vi "Compute slopes from compensate values.vi"(0 "SAVE_Aberrations Filter in":T4, 5 "FilteredSlopesX in":dbl[][](array[numeric]), 7 "FilteredSlopesY in":dbl[][](array[numeric]), 9 "Pupil":i32[][](array[numeric]), 11 "Dimensions_um":T1, 12 "SlopesX_fitting":cluster{"a":dbl, "b":dbl, "c":dbl}, 13 "SlopesY_fitting":cluster{"a":dbl, "b":dbl, "c":dbl}, 14 "Delta_um":T3) -> (6 "FilteredSlopesX out":dbl[][](array[numeric]), 8 "FilteredSlopesY out":dbl[][](array[numeric]))   [LabVIEW 2020]
uses:
  Point2Df.ctl
  General dimensions definition.ctl
  Point2D.ctl
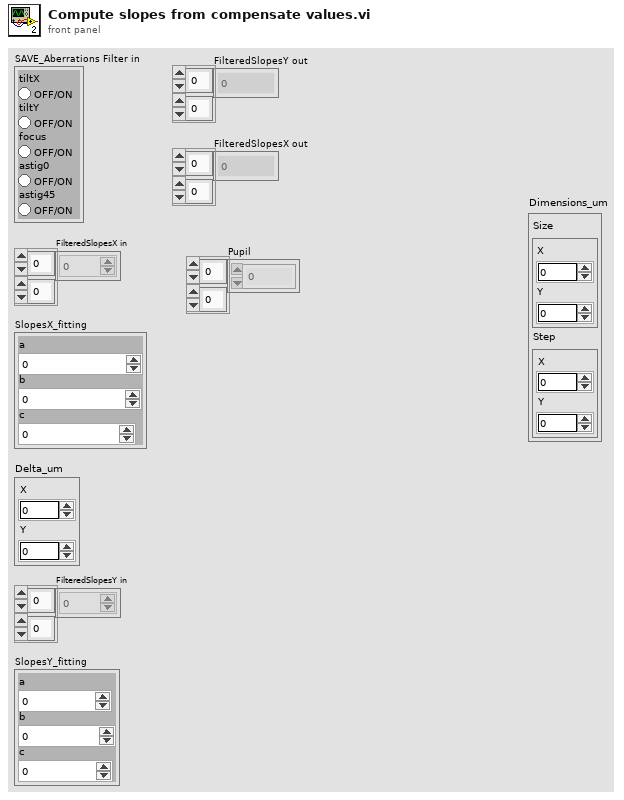
[diagram p1: front panel]
types:
  T1 = typedef "General dimensions definition.ctl" = cluster{"Size":T2, "Step":T3}
  T2 = typedef "Point2D.ctl" = cluster{"X":u32, "Y":u32}
  T3 = typedef "Point2Df.ctl" = cluster{"X":sgl, "Y":sgl}
  T4 = cluster{"tiltX":bool, "tiltY":bool, "focus":bool, "astig0":bool, "astig45":bool}
  T5 = cluster{"ax":dbl, "bx":dbl, "cx":dbl, "ay":dbl, "by":dbl, "cy":dbl, "Delta":T3}
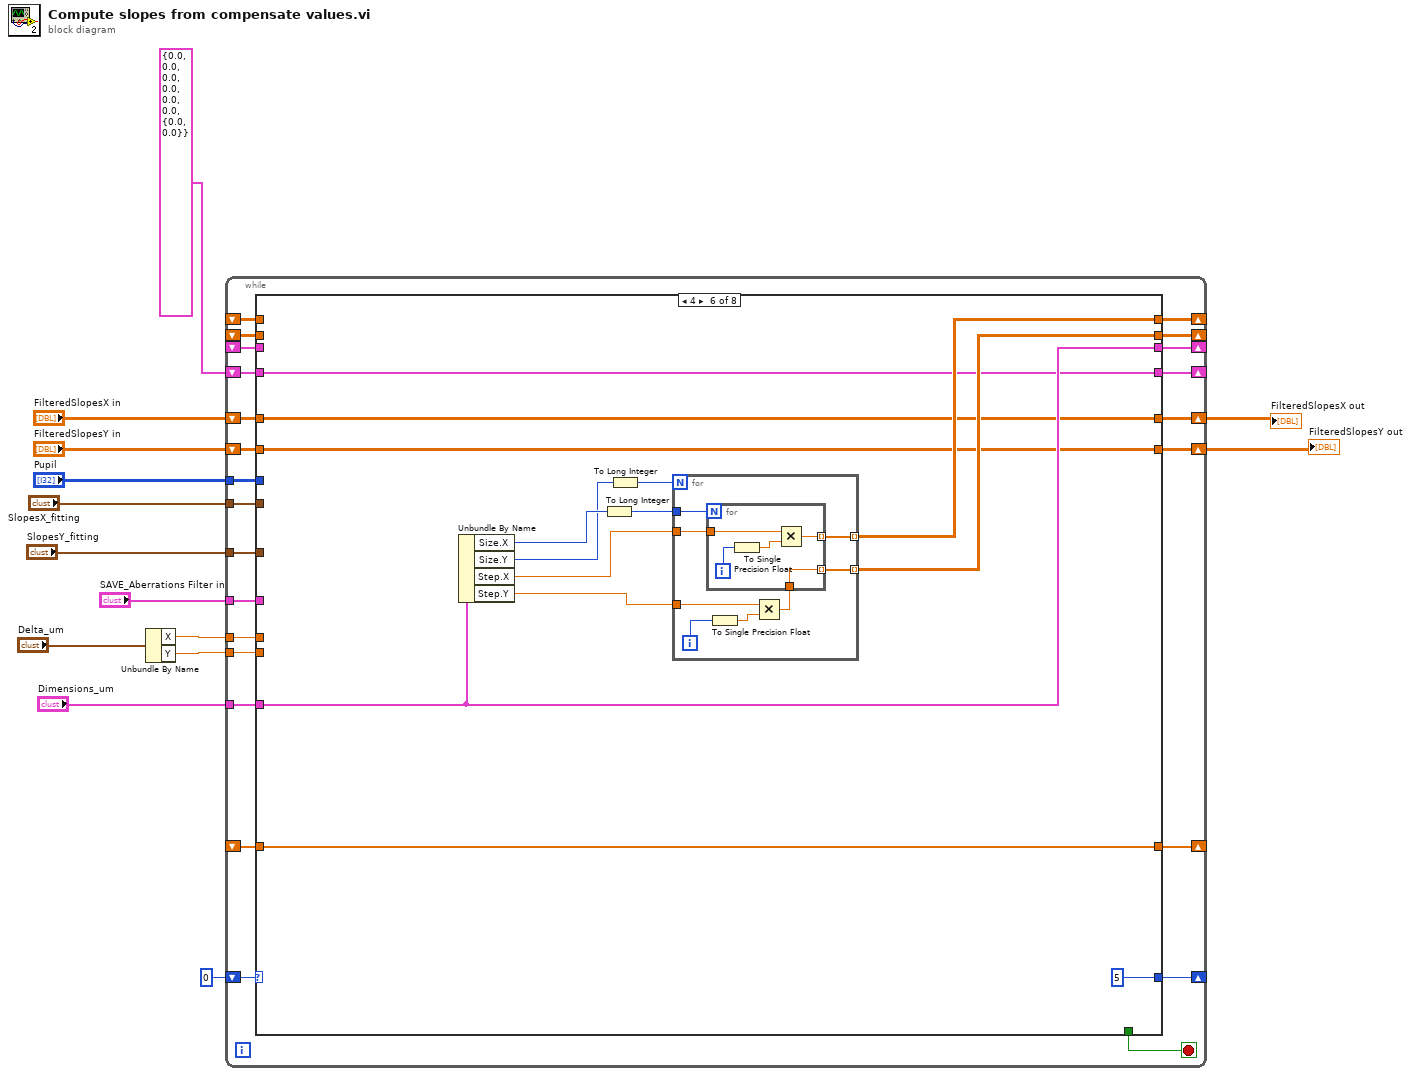
[diagram p0: block diagram]
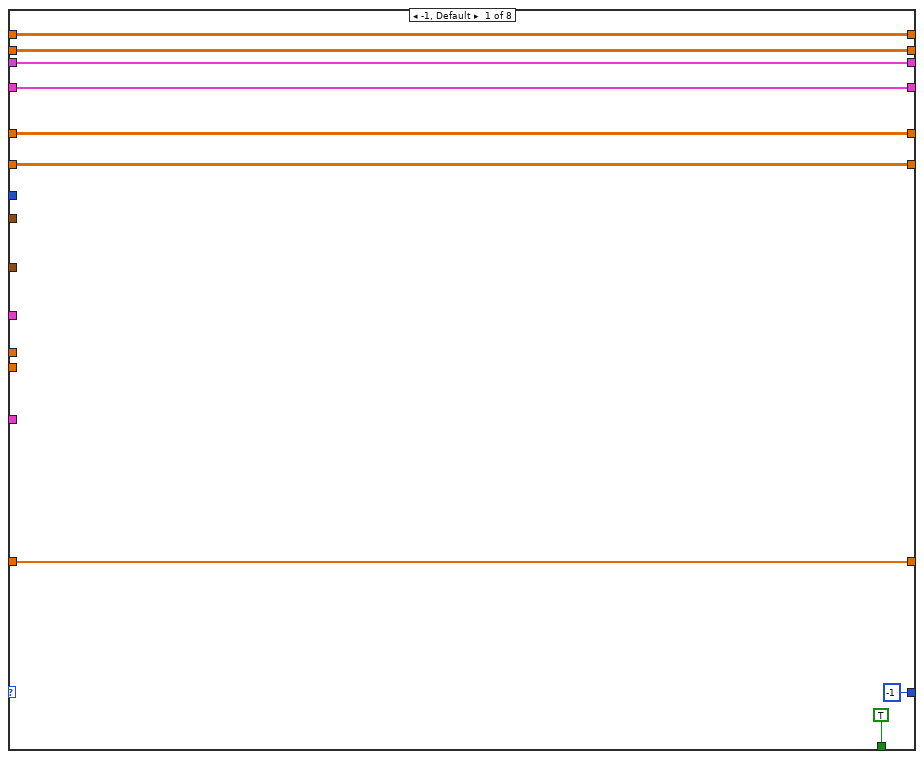
[diagram p2: hidden frame]
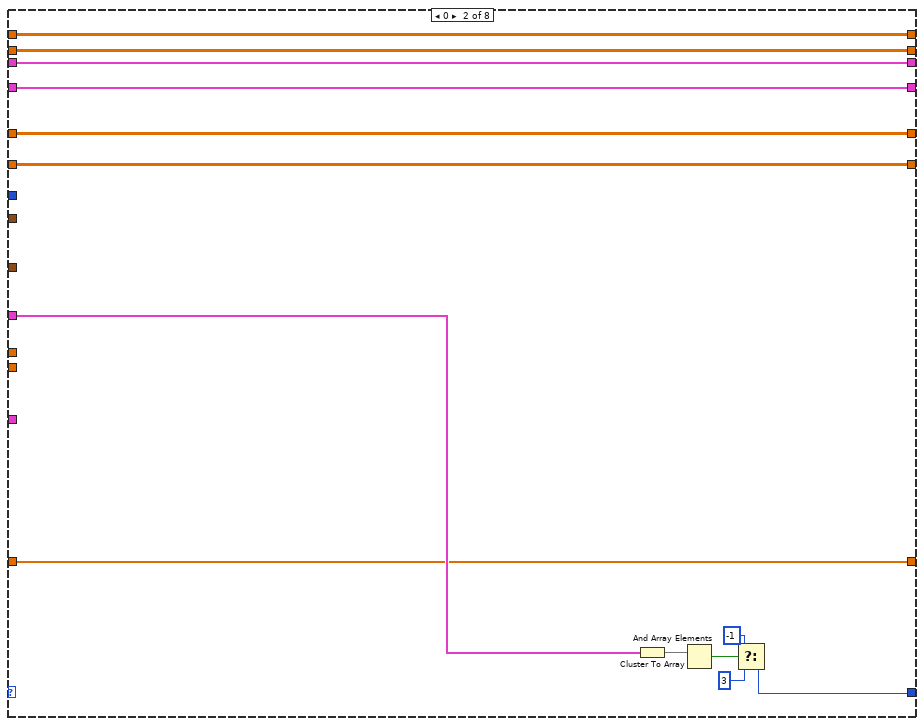
[diagram p3: hidden frame]
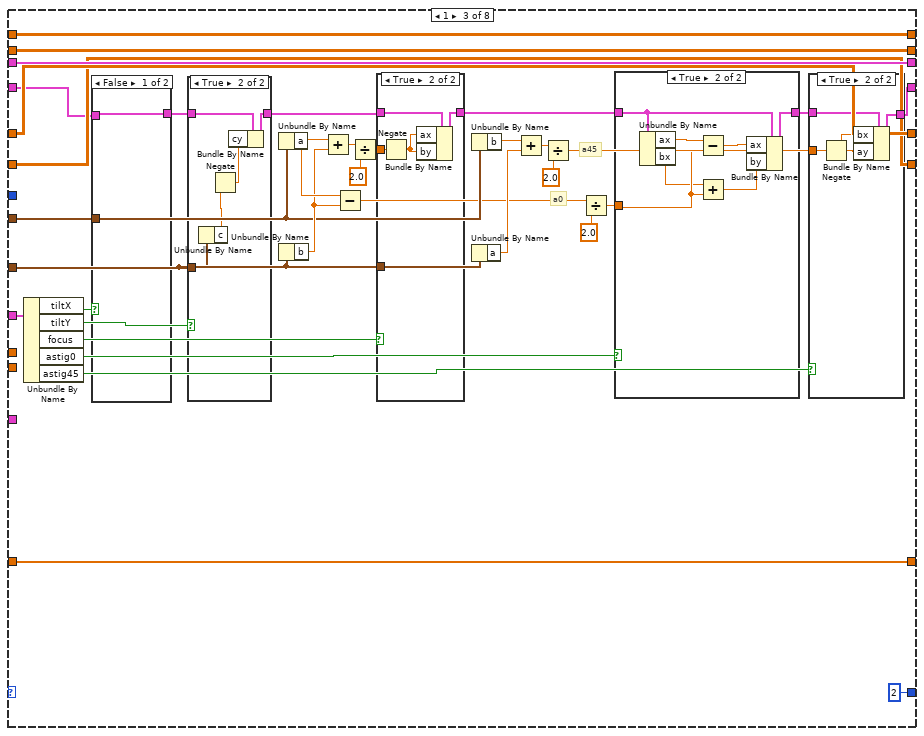
[diagram p4: hidden frame]
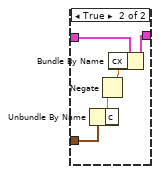
[diagram p9: hidden frame]
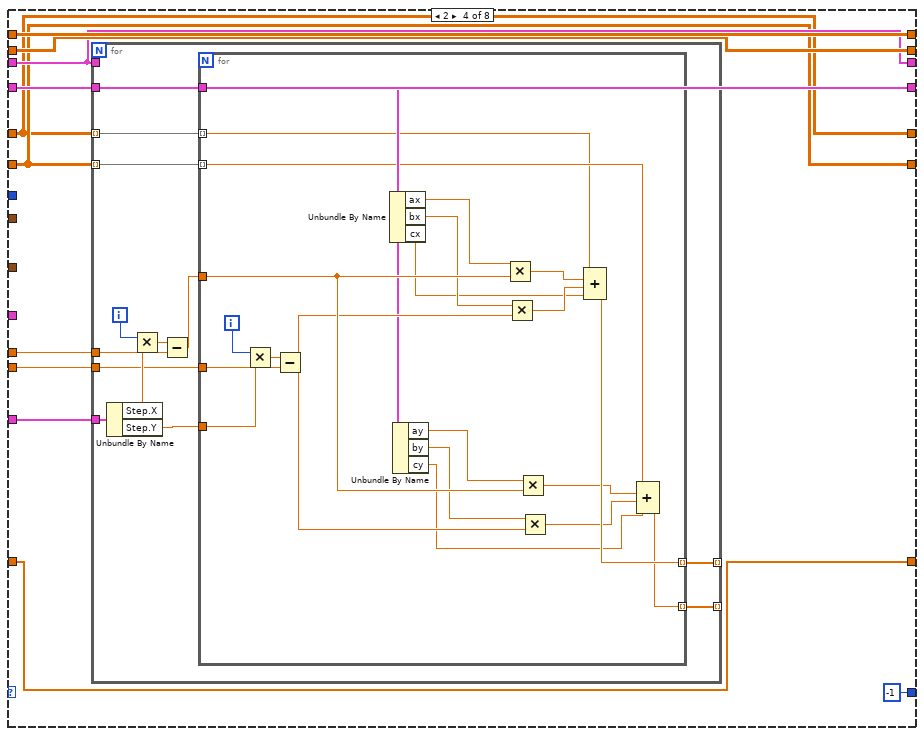
[diagram p10: hidden frame]
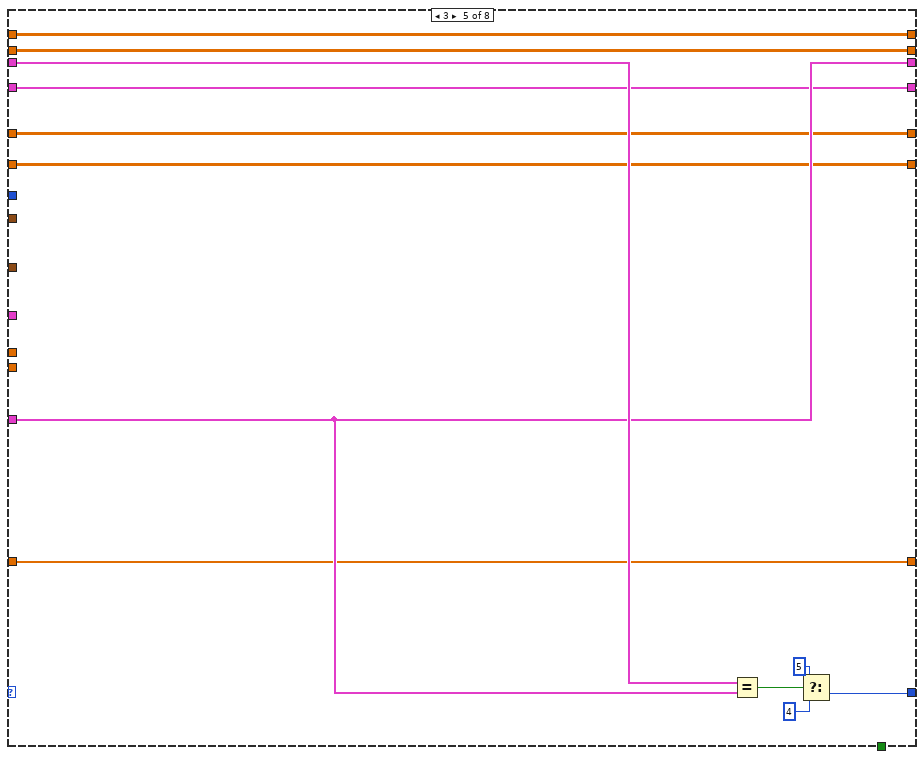
[diagram p11: hidden frame]
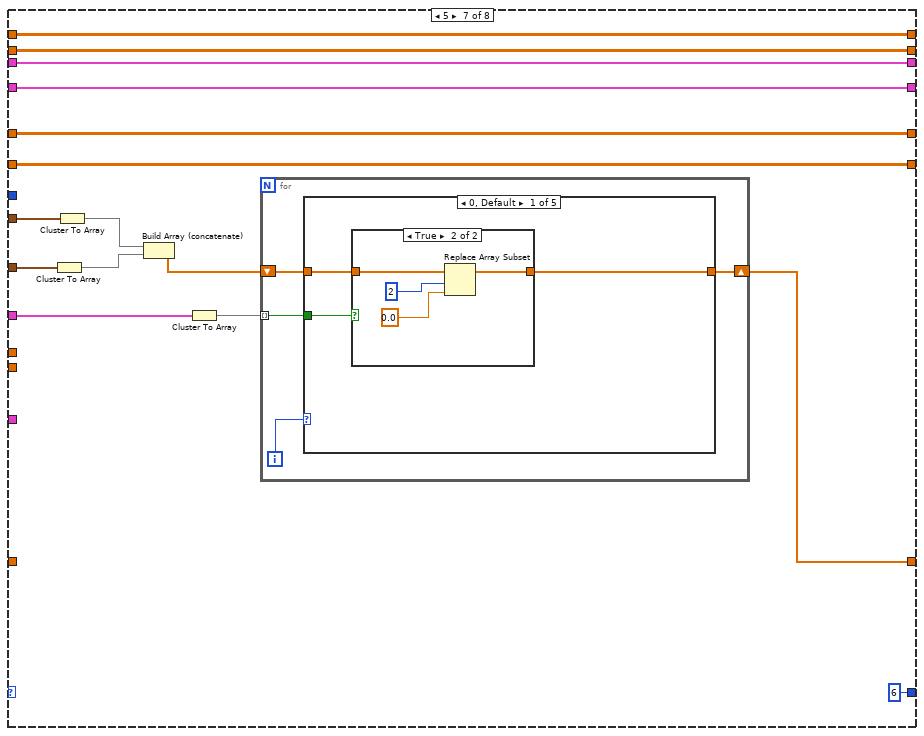
[diagram p12: hidden frame]
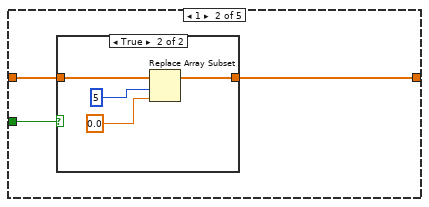
[diagram p14: hidden frame]
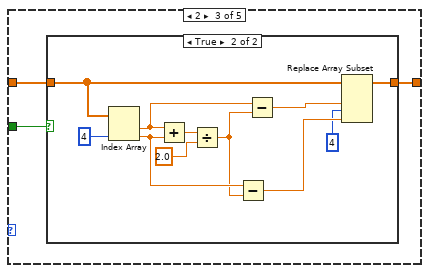
[diagram p16: hidden frame]
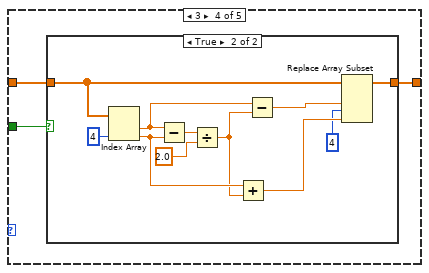
[diagram p18: hidden frame]
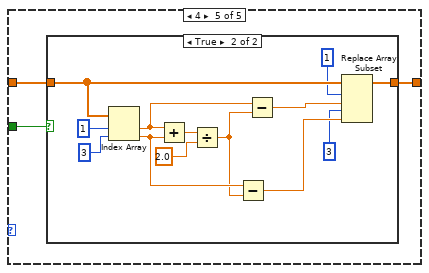
[diagram p20: hidden frame]
diagram:
  n1 = Unbundle By Name("Delta_um") -> ("X"=w3:sgl, "Y"=w2:sgl)
  n2 = while {
    tunnel: "SAVE_Aberrations Filter in" -> [w38]
    tunnel: "SlopesX_fitting" -> [w37]
    tunnel: "SlopesY_fitting" -> [w36]
    shift-right: [w33] -> _
    shift-left: 0 -> [w35]
    shift-right: [w19] -> w6
    shift-left: "FilteredSlopesX in" -> [w21]
    shift-right: [w18] -> w12
    shift-left: "FilteredSlopesY in" -> [w20]
    shift-right: [w34] -> _
    shift-left: T5 {"ax"=0.0, "bx"=0.0, "cx"=0.0, "ay"=0.0, "by"=0.0, "cy"=0.0, "Delta"={"X"=0.0, "Y"=0.0}} -> [w15]
    tunnel: "Dimensions_um" -> [w31]
    tunnel: w3 -> [w30]
    tunnel: w2 -> [w29]
    shift-right: [w27] -> _
    shift-left: _ -> [w28]
    shift-right: [w25] -> _
    shift-left: _ -> [w24]
    shift-right: [w26] -> _
    shift-left: _ -> [w23]
    shift-right: [w22] -> _
    shift-left: _ -> [w17]
    tunnel: "Pupil" -> [w16]
    stop <- w32 stop-if-true
    n3 = case shown="4" w35 {
      tunnel: w38 -> [_ w59 w94 _ _ _ w218 _]
      tunnel: w37 -> [_ _ w76 _ _ _ w217 _]
      tunnel: w36 -> [_ _ w77 _ _ _ w216 _]
      tunnel: [w39 w48 w61 w127 w170 w182 w209 w291] -> w34
      tunnel: [-1 w55 2 -1 w178 5 6 -1] -> w33
      tunnel: [TRUE _ _ _ _ _ _ _] -> w32
      tunnel: w31 -> [_ _ _ w135 w176 w189 _ _]
      tunnel: w30 -> [_ _ _ w134 _ _ _ w294]
      tunnel: w29 -> [_ _ _ w133 _ _ _ w292]
      tunnel: w28 -> [w43 w52 w66 w128 w177 _ w220 w302]
      tunnel: [w43 w52 w66 w128 w176 w189 w220 w302] -> w27
      tunnel: [w44 w53 w67 w130 w174 w188 w221 w293] -> w26
      tunnel: [w45 w54 w68 w131 w175 w187 w222 w297] -> w25
      tunnel: w24 -> [w45 w54 w68 w131 w175 _ w222 w297]
      tunnel: w23 -> [w44 w53 w67 w130 w174 _ w221 w293]
      tunnel: [w40 w49 w63 w129 w171 w183 w212 w295] -> w22
      tunnel: w21 -> [w42 w51 w65 w125 w173 w185 w211 w301]
      tunnel: w20 -> [w41 w50 w64 w126 w172 w184 w210 w300]
      tunnel: [w42 w51 w65 w125 w173 w185 w211 w299] -> w19
      tunnel: [w41 w50 w64 w126 w172 w184 w210 w298] -> w18
      tunnel: w17 -> [w40 w49 w63 w129 w171 w183 _ w295]
      tunnel: w16 -> [_ _ _ _ _ _ _ w296]
      tunnel: w15 -> [w39 w48 w62 w127 w170 w182 w209 w291]
      frame -1, Default {
      }
      frame 0 {
        n4 = Cluster To Array(cluster=w59) -> (array=w60:bool[])
        n5 = And Array Elements(Boolean array=w60) -> (logical AND=w57:bool)
        n6 = Select(t=-1, s=w57, f=3) -> (s? t:f=w55:i32)
      }
      frame 1 {
        # "a45"
        # "a0"
        n7 = Unbundle By Name(w94) -> ("tiltX"=w93:bool, "tiltY"=w91:bool, "focus"=w86:bool, "astig0"=w85:bool, "astig45"=w72:bool)
        n8 = case shown="False" w93 {
          tunnel: [w119 w124] -> w92
          tunnel: w76 -> [_ w122]
          tunnel: w62 -> [w119 w120]
          frame False {
          }
          frame True {
            n9 = Unbundle By Name(w122) -> ("c"=w123:dbl)
            n10 = Negate(x=w123) -> (-x=w121:dbl)
            n11 = Bundle By Name(cluster=w120, "cx"=w121) -> (w124:T5)
          }
        }
        n12 = case shown="True" w91 {
          tunnel: w92 -> [w113 w118]
          tunnel: [w113 w117] -> w90
          tunnel: w77 -> [_ w116]
          frame False {
          }
          frame True {
            n13 = Unbundle By Name(w116) -> ("c"=w115:dbl)
            n14 = Negate(x=w115) -> (-x=w114:dbl)
            n15 = Bundle By Name(cluster=w118, "cy"=w114) -> (w117:T5)
          }
        }
        n16 = Unbundle By Name(w76) -> ("a"=w83:dbl)
        n17 = Unbundle By Name(w77) -> ("b"=w82:dbl)
        n18 = Add(x=w83, y=w82) -> (x+y=w88:dbl)
        n19 = Subtract(x=w83, y=w82) -> (x-y=w74:dbl)
        n20 = Divide(x=w88, y=2.0) -> (x/y=w87:dbl)
        n21 = case shown="True" w86 {
          tunnel: w90 -> [w108 w112]
          tunnel: [w108 w111] -> w84
          tunnel: w77 -> [_ _]
          tunnel: w87 -> [_ w110]
          frame False {
          }
          frame True {
            n22 = Negate(x=w110) -> (-x=w109:dbl)
            n23 = Bundle By Name(cluster=w112, "ax"=w109, "by"=w109) -> (w111:T5)
          }
        }
        n24 = Unbundle By Name(w76) -> ("b"=w80:dbl)
        n25 = Unbundle By Name(w77) -> ("a"=w81:dbl)
        n26 = Add(x=w80, y=w81) -> (x+y=w79:dbl)
        n27 = Divide(x=w79, y=2.0) -> (x/y=w71:dbl)
        n28 = Divide(x=w74, y=2.0) -> (x/y=w73:dbl)
        n29 = case shown="True" w85 {
          tunnel: w84 -> [w100 w106]
          tunnel: [w100 w107] -> w70
          tunnel: w73 -> [_ w104]
          frame False {
          }
          frame True {
            n30 = Unbundle By Name(w106) -> ("ax"=w102:dbl, "bx"=w101:dbl)
            n31 = Subtract(x=w102, y=w104) -> (x-y=w105:dbl)
            n32 = Add(x=w101, y=w104) -> (x+y=w103:dbl)
            n33 = Bundle By Name(cluster=w106, "ax"=w105, "by"=w103) -> (w107:T5)
          }
        }
        n34 = case shown="True" w72 {
          tunnel: w71 -> [_ w98]
          tunnel: w70 -> [w95 w99]
          tunnel: [w95 w96] -> w61
          frame False {
          }
          frame True {
            n35 = Negate(x=w98) -> (-x=w97:dbl)
            n36 = Bundle By Name(cluster=w99, "bx"=w97, "ay"=w97) -> (w96:T5)
          }
        }
      }
      frame 2 {
        n37 = for {
          tunnel: w135 -> [w147]
          tunnel: w134 -> [w144]
          tunnel: w133 -> [w142]
          tunnel: [w140] -> _ mode=indexing
          tunnel: [w139] -> _ mode=indexing
          tunnel: w128 -> [_]
          tunnel: w127 -> [w138]
          tunnel: w126 -> [w137] mode=indexing
          tunnel: w125 -> [w136] mode=indexing
          i -> [w148]
          n38 = Unbundle By Name(w147) -> ("Step.X"=w146:sgl, "Step.Y"=w143:sgl)
          n39 = Multiply(x=w148, y=w146) -> (x*y=w145:sgl)
          n40 = Subtract(x=w145, y=w144) -> (x-y=w141:sgl)
          n41 = for {
            tunnel: w143 -> [w167]
            tunnel: w142 -> [w166]
            tunnel: w141 -> [w160]
            tunnel: [w163] -> w140 mode=indexing
            tunnel: [w158] -> w139 mode=indexing
            tunnel: w138 -> [w157]
            tunnel: w137 -> [w150] mode=indexing
            tunnel: w136 -> [w149] mode=indexing
            i -> [w168]
            n42 = Multiply(x=w168, y=w167) -> (x*y=w169:sgl)
            n43 = Subtract(x=w169, y=w166) -> (x-y=w159:sgl)
            n44 = Unbundle By Name(w157) -> ("ax"=w156:dbl, "bx"=w155:dbl, "cx"=w154:dbl)
            n45 = Unbundle By Name(w157) -> ("ay"=w153:dbl, "by"=w152:dbl, "cy"=w151:dbl)
            n46 = Multiply(x=w156, y=w160) -> (x*y=w165:dbl)
            n47 = Multiply(x=w155, y=w159) -> (x*y=w164:dbl)
            n48 = Multiply(x=w153, y=w160) -> (x*y=w161:dbl)
            n49 = Multiply(x=w152, y=w159) -> (x*y=w162:dbl)
            n50 = Compound Arithmetic op=ADD(w149, w165, w164, w154) -> (w163:dbl)
            n51 = Compound Arithmetic op=ADD(w150, w161, w162, w151) -> (w158:dbl)
          }
        }
      }
      frame 3 {
        n52 = Equal?(x=w177, y=w176) -> (x = y?=w179:bool)
        n53 = Select(t=5, s=w179, f=4) -> (s? t:f=w178:i32)
      }
      frame 4 {
        n54 = Unbundle By Name(w189) -> ("Size.X"=w195:u32, "Size.Y"=w192:u32, "Step.X"=w193:sgl, "Step.Y"=w190:sgl)
        n55 = To Long Integer(number=w195) -> (32bit integer=w194:i32)
        n56 = To Long Integer(number=w192) -> (32bit integer=w191:i32)
        n57 = for {
          N: w191 -> [_]
          tunnel: w194 -> [w203]
          tunnel: w193 -> [w202]
          tunnel: [w201] -> w187 mode=indexing
          tunnel: w190 -> [w198]
          tunnel: [w196] -> w188 mode=indexing
          i -> [w199]
          n58 = To Single Precision Float(number=w199) -> (single precision float=w200:sgl)
          n59 = Multiply(x=w198, y=w200) -> (x*y=w197:sgl)
          n60 = for {
            N: w203 -> [_]
            tunnel: w202 -> [w208]
            tunnel: [w205] -> w201 mode=indexing
            tunnel: w197 -> [w204]
            tunnel: [w204] -> w196 mode=indexing
            i -> [w207]
            n61 = To Single Precision Float(number=w207) -> (single precision float=w206:sgl)
            n62 = Multiply(x=w208, y=w206) -> (x*y=w205:sgl)
          }
        }
      }
      frame 5 {
        n63 = Cluster To Array(cluster=w216) -> (array=w214:dbl[])
        n64 = Cluster To Array(cluster=w217) -> (array=w215:dbl[])
        n65 = Build Array (concatenate)(w215, w214) -> (w213:dbl[])
        n66 = Cluster To Array(cluster=w218) -> (array=w219:bool[])
        n67 = for {
          tunnel: w219 -> [w227] mode=indexing
          shift-right: [w225] -> w212
          shift-left: w213 -> [w226]
          i -> [w224]
          n68 = case shown="0, Default" w224 {
            tunnel: w227 -> [w230 w238 w246 w261 w276]
            tunnel: w226 -> [w229 w237 w245 w260 w275]
            tunnel: [w228 w236 w244 w259 w274] -> w225
            frame 0, Default {
              n69 = case shown="True" w230 {
                tunnel: w229 -> [w231 w235]
                tunnel: [w231 w234] -> w228
                frame False {
                }
                frame True {
                  n70 = Replace Array Subset(array=w235, new element=sgl 0.0 ("new element/subarray"), index=2) -> (w234:dbl[])
                }
              }
            }
            frame 1 {
              n71 = case shown="True" w238 {
                tunnel: w237 -> [w239 w243]
                tunnel: [w239 w242] -> w236
                frame False {
                }
                frame True {
                  n72 = Replace Array Subset(array=w243, new element=sgl 0.0 ("new element/subarray"), index=5) -> (w242:dbl[])
                }
              }
            }
            frame 2 {
              n73 = case shown="True" w246 {
                tunnel: w245 -> [w247 w248]
                tunnel: [w247 w258] -> w244
                frame False {
                }
                frame True {
                  n74 = Index Array(array=w248, index #2=4 ("index")) -> (element #1=w254:dbl, element #2=w253:dbl)  [unwired: 1 in]
                  n75 = Add(x=w254, y=w253) -> (x+y=w256:dbl)
                  n76 = Divide(x=w256, y=sgl 2.0) -> (x/y=w252:dbl)
                  n77 = Subtract(x=w253, y=w252) -> (x-y=w250:dbl)
                  n78 = Subtract(x=w254, y=w252) -> (x-y=w251:dbl)
                  n79 = Replace Array Subset(array=w248, new element #1=w251, new element #2=w250, index #2=4 ("index")) -> (w258:dbl[])  [unwired: 1 in]
                }
              }
            }
            frame 3 {
              n80 = case shown="True" w261 {
                tunnel: w260 -> [w262 w263]
                tunnel: [w262 w273] -> w259
                frame False {
                }
                frame True {
                  n81 = Index Array(array=w263, index #2=4 ("index")) -> (element #1=w269:dbl, element #2=w268:dbl)  [unwired: 1 in]
                  n82 = Subtract(x=w269, y=w268) -> (x-y=w271:dbl)
                  n83 = Divide(x=w271, y=sgl 2.0) -> (x/y=w267:dbl)
                  n84 = Add(x=w268, y=w267) -> (x+y=w265:dbl)
                  n85 = Subtract(x=w269, y=w267) -> (x-y=w266:dbl)
                  n86 = Replace Array Subset(array=w263, new element #1=w266, new element #2=w265, index #2=4 ("index")) -> (w273:dbl[])  [unwired: 1 in]
                }
              }
            }
            frame 4 {
              n87 = case shown="True" w276 {
                tunnel: w275 -> [w277 w280]
                tunnel: [w277 w290] -> w274
                frame False {
                }
                frame True {
                  n88 = Index Array(array=w280, index #1=1 ("index"), index #2=3 ("index")) -> (element #1=w286:dbl, element #2=w285:dbl)
                  n89 = Add(x=w286, y=w285) -> (x+y=w288:dbl)
                  n90 = Divide(x=w288, y=sgl 2.0) -> (x/y=w284:dbl)
                  n91 = Subtract(x=w285, y=w284) -> (x-y=w282:dbl)
                  n92 = Subtract(x=w286, y=w284) -> (x-y=w283:dbl)
                  n93 = Replace Array Subset(array=w280, new element #1=w283, index #1=1 ("index"), new element #2=w282, index #2=3 ("index")) -> (w290:dbl[])
                }
              }
            }
          }
        }
      }
      frame 6 {
        n94 = for {
          tunnel: w301 -> [w313] mode=indexing
          tunnel: w300 -> [w312] mode=indexing
          tunnel: w296 -> [w311] mode=indexing
          tunnel: w295 -> [w310]
          tunnel: [w309] -> w299 mode=indexing
          tunnel: [w308] -> w298 mode=indexing
          tunnel: w297 -> [w307] mode=indexing
          tunnel: w294 -> [w306]
          tunnel: w293 -> [w305] mode=indexing
          tunnel: w292 -> [w304]
          n95 = for {
            tunnel: w313 -> [w322] mode=indexing
            tunnel: w312 -> [w320] mode=indexing
            tunnel: w311 -> [w323] mode=indexing
            tunnel: w310 -> [w321]
            tunnel: [w319] -> w309 mode=indexing
            tunnel: [w318] -> w308 mode=indexing
            tunnel: w307 -> [w317] mode=indexing
            tunnel: w306 -> [w316]
            tunnel: w305 -> [w315] mode=indexing
            tunnel: w304 -> [w314]
            n96 = case shown="1" w323 {
              tunnel: w322 -> [_ w341]
              tunnel: w321 -> [_ w347]
              tunnel: w320 -> [_ w339]
              tunnel: [w324 w332] -> w319
              tunnel: [w324 w331] -> w318
              tunnel: w317 -> [_ w330]
              tunnel: w316 -> [_ w329]
              tunnel: w315 -> [_ w327]
              tunnel: w314 -> [_ w326]
              frame 0, Default {
                w324 = sgl nan
              }
              frame 1 {
                n97 = Subtract(x=w327, y=w326) -> (x-y=w325:sgl)
                n98 = Subtract(x=w330, y=w329) -> (x-y=w328:sgl)
                n99 = Index Array(array=w347) -> (element #1=w346:dbl, element #2=w345:dbl, element #3=w342:dbl, element #4=w336:dbl, element #5=w335:dbl, element #6=w334:dbl)  [unwired: 6 in]
                n100 = Multiply(x=w328, y=w336) -> (x*y=w338:dbl)
                n101 = Multiply(x=w325, y=w335) -> (x*y=w337:dbl)
                n102 = Multiply(x=w328, y=w346) -> (x*y=w343:dbl)
                n103 = Multiply(x=w325, y=w345) -> (x*y=w344:dbl)
                n104 = Compound Arithmetic op=ADD(w338, w337, w334) -> (w333:dbl)
                n105 = Compound Arithmetic op=ADD(w343, w344, w342) -> (w340:dbl)
                n106 = Add(x=w341, y=w340) -> (x+y=w332:dbl)
                n107 = Add(x=w339, y=w333) -> (x+y=w331:dbl)
              }
            }
          }
        }
      }
    }
  }
  "FilteredSlopesY out" <- w12
  "FilteredSlopesX out" <- w6
